vi "Create Redirect.vi"(8 "error in (no error)":errorcluster, 9 "Force GET? (F)":bool, 10 "Permanent? (F)":bool, 11 "Redirect URI":refnum<class "URI.lvclass">) -> (0 "error out":errorcluster, 3 "Redirect Response out":refnum<class "Redirect Response.lvclass">)   [LabVIEW 2020, in "HTTP Utils.lvlib" / "Redirect Response.lvclass"]
uses:
  Redirect Response.lvclass
  C:/dev/lv20CE/relink/lv-http-util/HTTP Utils/Response/Response.lvclass
  Redirect Response.lvclass/Redirect Response.ctl
  Response/Response.lvclass
  C:/dev/lv20CE/relink/lv-http-util/HTTP Utils/Redirect Response/Redirect Response.lvclass
  lv-uri/URI/URI/URI.lvclass
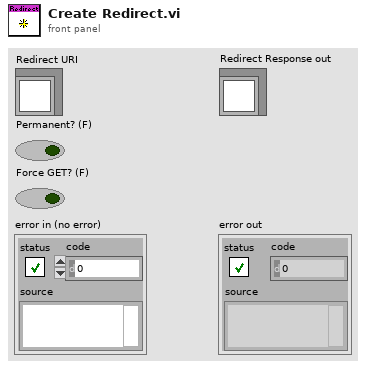
[diagram p1: front panel]
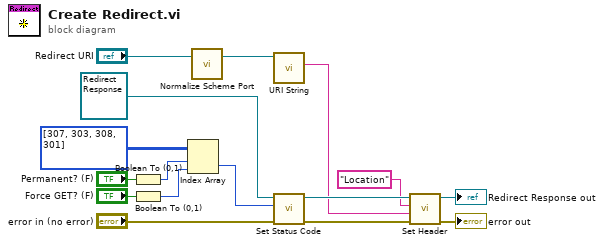
[diagram p0: block diagram]
diagram:
  n1 = Boolean To (0,1)(Boolean="Permanent? (F)") -> (0, 1=w5:i16)
  n2 = Boolean To (0,1)(Boolean="Force GET? (F)") -> (0, 1=w4:i16)
  n3 = Index Array(array=u16[][] [[307, 303], [308, 301]], index (row)=w5, index (col)=w4) -> (element=w3:u16)
  n4 = call "Normalize Scheme Port.vi"("URI in"="Redirect URI") -> ("URI out"=w1:refnum<class "URI.lvclass">)  [unwired: 6 in]
  n5 = call "URI String.vi"("URI in"=w1) -> ("URI String"=w10:string)  [unwired: 9 in, 1 out]
  n6 = call "Set Status Code.vi"("error in (no error)"="error in (no error)", "Status Code"=w3, "Response in"=refnum<class "Redirect Response.lvclass"> refnum ("Redirect Response out")) -> ("error out"=w14:errorcluster, "Response out"=w15:refnum<class "Redirect Response.lvclass">)  [unwired: 7 in]
  n7 = call "Set Header.vi"("error in (no error)"=w14, "Value"=w10, "Header"="Location", "Response in"=w15) -> ("error out"=→"error out":errorcluster, "Response out"=→"Redirect Response out":refnum<class "Redirect Response.lvclass">)  [unwired: 5 in, 1 out]
